vi "Control Mode.vi"(7 "Communication Address (0)":i16 max=254 format="%x", 8 "error in (no error)":errorcluster, 9 "Enable Local Control (T: On)":bool=TRUE, 10 "Enable Remote Mode (F: Off)":bool, 11 "VISA resource name":refnum<visa-resource-name>) -> (0 "error out":errorcluster, 3 "VISA resource name out":refnum<visa-resource-name>)   [LabVIEW 2019, in "BK Precision 178XB Series.lvlib"]
doc: "This VI sets the mode of operation. <b>Remote mode</b> must be set to ON in order to control DC load over serial interface. If OFF, control operations can only be done from the physical front panel of the load. When <b>Local Control</b> is (F:OFF), all front panel keys will be disabled and changing to local mode from front panel will also be disabled. Use this VI if the instrument must strictly be controlled remotely without interruption from front panel keys."
uses:
  BK Precision 178XB Series.lvlib
panel:
  # "(c) 2009 B&K PRECISION CORPORATION.  ALL RIGHTS RESERVED."
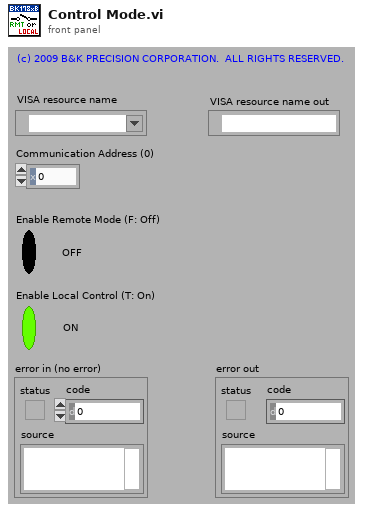
[diagram p1: front panel]
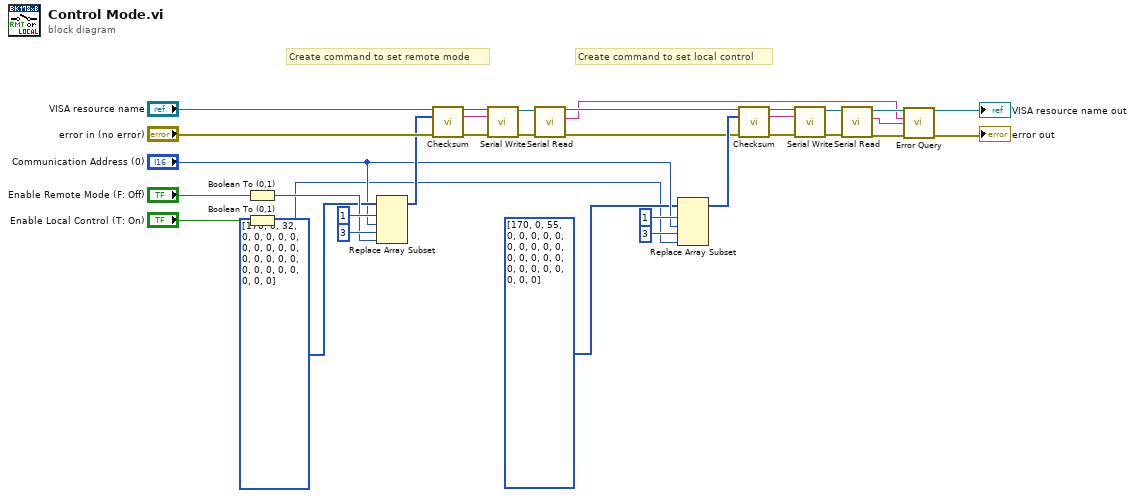
[diagram p0: block diagram]
diagram:
  # "Create command to set local control"
  # "Create command to set remote mode"
  n1 = Boolean To (0,1)(Boolean="Enable Remote Mode (F: Off)") -> (0, 1=w9:i16)
  n2 = Boolean To (0,1)(Boolean="Enable Local Control (T: On)") -> (0, 1=w1:i16)
  n3 = Replace Array Subset(array=i16[] [170, 0, 32, 0, 0, 0, 0, 0, 0, 0, 0, 0, 0, 0, 0, 0, 0, 0, 0, 0, 0, 0, 0, 0, 0, 0], new element #1="Communication Address (0)", index #1=1, new element #2=w9, index #2=3) -> (w7:i16[])
  n4 = call "Checksum.vi"("VISA resource name"="VISA resource name", "Command Frame Array"=w7, "error in (no error)"="error in (no error)") -> ("VISA resource name out"=w26:refnum<visa-resource-name>, "Output String"=w25:string, "error out"=w27:errorcluster)  [unwired: 8 in, 2 out]
  n5 = call "Serial Write.vi"("error in (no error)"=w27, "Input Command Frame"=w25, "VISA resource name"=w26) -> ("error out"=w32:errorcluster, "VISA resource name out"=w33:refnum<visa-resource-name>)  [unwired: 6 in, 1 out]
  n6 = call "Serial Read.vi"("error in (no error)"=w32, "VISA resource name"=w33) -> ("error out"=w15:errorcluster, "Read Buffer"=w14:string, "VISA resource name out"=w16:refnum<visa-resource-name>)  [unwired: 7 in]
  n7 = Replace Array Subset(array=i16[] [170, 0, 55, 0, 0, 0, 0, 0, 0, 0, 0, 0, 0, 0, 0, 0, 0, 0, 0, 0, 0, 0, 0, 0, 0, 0], new element #1="Communication Address (0)", index #1=1, new element #2=w1, index #2=3) -> (w22:i16[])
  n8 = call "Checksum.vi"("VISA resource name"=w16, "Command Frame Array"=w22, "error in (no error)"=w15) -> ("VISA resource name out"=w20:refnum<visa-resource-name>, "Output String"=w19:string, "error out"=w21:errorcluster)  [unwired: 8 in, 2 out]
  n9 = call "Serial Write.vi"("error in (no error)"=w21, "Input Command Frame"=w19, "VISA resource name"=w20) -> ("error out"=w23:errorcluster, "VISA resource name out"=w24:refnum<visa-resource-name>)  [unwired: 6 in, 1 out]
  n10 = call "Serial Read.vi"("error in (no error)"=w23, "VISA resource name"=w24) -> ("error out"=w18:errorcluster, "Read Buffer"=w13:string, "VISA resource name out"=w17:refnum<visa-resource-name>)  [unwired: 7 in]
  n11 = call "Error Query.vi"("VISA resource name"=w17, "Input Read Buffer 1"=w14, "Input Read Buffer 2"=w13, "error in (no error)"=w18) -> ("VISA resource name out"=→"VISA resource name out":refnum<visa-resource-name>, "error out"=→"error out":errorcluster)  [unwired: 6 in, 4 out]
